vi "选择设备.vi"() -> (0 "boot?":bool, 3 "路径":path)   [LabVIEW 2020]
panel:
  in  "列表框":i32(listbox)
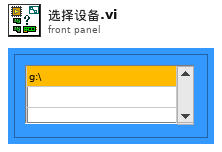
[diagram p1: front panel]
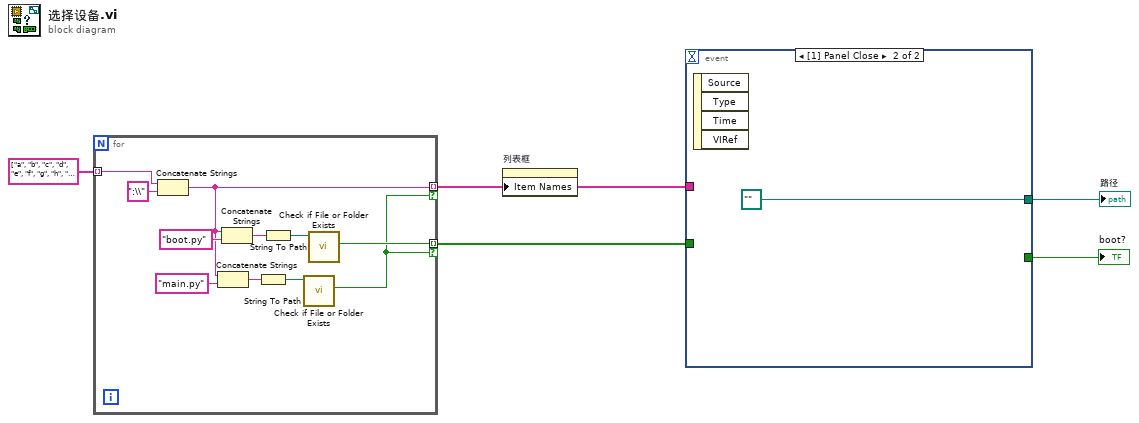
[diagram p0: block diagram]
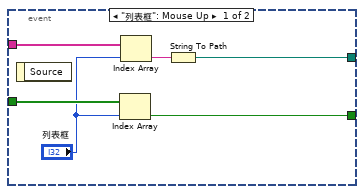
[diagram p2: hidden frame]
diagram:
  n1 = for {
    tunnel: string[] ["a", "b", "c", "d", "e", "f", "g", "h", "i", "j", "k", "l", "m", "n", "o", "p", "q", "r", "s", "t", "u", "v", "w", "x", "y", "z"] -> [w16] mode=indexing
    tunnel: [w8] -> w4 mode=indexing if=w6
    tunnel: [w7] -> w2 mode=indexing if=w6
    n2 = Concatenate Strings(w16, ":\\" ("字符串")) -> (w8:string)
    n3 = Concatenate Strings(w8, "main.py" ("字符串")) -> (w10:string)
    n4 = Concatenate Strings(w8, "boot.py" ("字符串")) -> (w12:string)
    n5 = String To Path(string=w10) -> (path=w9:path)
    n6 = String To Path(string=w12) -> (path=w14:path)
    n7 = call <vilib>:"Check if File or Folder Exists.vi"("path"=w9) -> ("file or folder exists?"=w6:bool)  [unwired: 8 in, 2 out]
    n8 = call <vilib>:"Check if File or Folder Exists.vi"("path"=w14) -> ("file or folder exists?"=w7:bool)  [unwired: 8 in, 2 out]
  }
  n9 = property on="列表框" class="LstBox (strict)"("Item Names"=w4) -> ()  [unwired: 2 in, 2 out]
  n10 = event shown="[1] Panel Close" {
    selector: _ -> [_ _]
    dyn-events: _ -> [_ _]
    timeout: _ -> [_ _]
    tunnel: w4 -> [w22 _]
    tunnel: [w20 path ""] -> w3
    tunnel: w2 -> [w19 _]
    tunnel: [w17 _] -> w1
    event "列表框": Mouse Up {
      n11 = event-data() -> ()  [unwired: 1 in, 1 out]
      n12 = Index Array(array=w19, index="列表框") -> (element=w17:bool)
      n13 = Index Array(array=w22, index="列表框") -> (element=w21:string)
      n14 = String To Path(string=w21) -> (path=w20:path)
    }
    event Panel Close {
      n15 = event-data() -> ()  [unwired: 1 in, 4 out]
    }
  }
  "路径" <- w3
  "boot?" <- w1
